vi "LTS60_TCP_Set_Relay_1.vi"(8 "error in (no error)":errorcluster, 10 "Beam":bool, 11 "connection ID":refnum<k5>) -> (0 "error out":errorcluster, 2 "Beam out":bool, 3 "connection ID out":refnum<k5>)   [LabVIEW 2019]
panel:
  out "data out":string
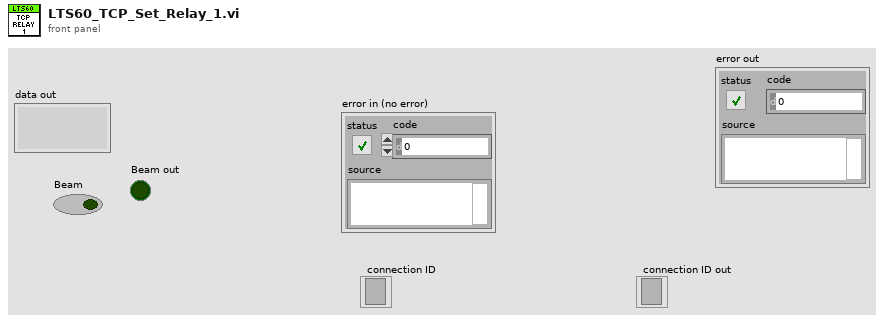
[diagram p1: front panel]
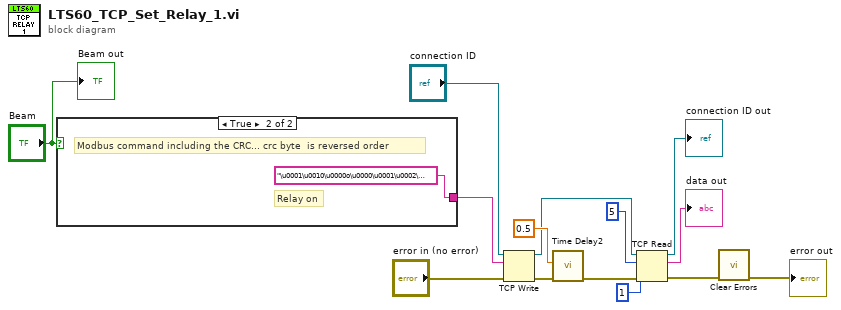
[diagram p0: block diagram]
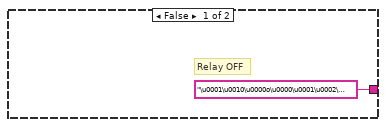
[diagram p2: hidden frame]
diagram:
  n1 = case shown="True" "Beam" {
    tunnel: ["\u0001\u0010\u0000o\u0000\u0001\u0002\u0000\u0000¯\u000f" ("write buffer") "\u0001\u0010\u0000o\u0000\u0001\u0002\u0000\u0001nÏ" ("write buffer")] -> w14
    frame False {
      # "Relay OFF"
    }
    frame True {
      # "Modbus command including the CRC... crc byte  is reversed order"
      # "Relay on"
    }
  }
  n2 = TCP Write(connection ID="connection ID", data in=w14, error in (no error)="error in (no error)") -> (connection ID out=w10:refnum<k5>, error out=w13:errorcluster)  [unwired: 1 in, 1 out]
  n3 = call "Time Delay2"("error in (no error)"=w13, "Delay Time (s)"=0.5) -> ("error out"=w11:errorcluster)  [unwired: 9 in]
  n4 = TCP Read(connection ID=w10, bytes to read=5, error in (no error)=w11, 9:1 ("timeout ms (25000)")) -> (connection ID out=→"connection ID out":refnum<k5>, data out=→"data out":string, error out=w2:errorcluster)  [unwired: 1 in]
  n5 = call <vilib>:"Clear Errors.vi"("error in (no error)"=w2) -> ("error out"=→"error out":errorcluster)  [unwired: 5 in, 1 out]
  "Beam out" <- "Beam"
